vi "MDO_video_analyzer.vi"() -> ()   [LabVIEW 2012]
uses:
  controls/Video_analizer_stats.ctl
  <vilib>/vision/Avi.llb/IMAQ AVI2 Codec Path.ctl
panel:
  out "Image":T1(plugin-control) caption="300В-пуск-1.avi"
  in  "Save image":bool
  in  "Enum":enum16{"Осциллограммы", "ВАХ"}(ring)=enum."ВАХ"
  in  "Load DAQ Data":bool
  in  "Load Video":bool
  in  "Frame Forward":bool
  in  "Frame Back":bool
  in  "Settings Button":bool
  in  "Play Button":bool
  in  "Slide":u32(slide) max=200 scale=0.0..200.0
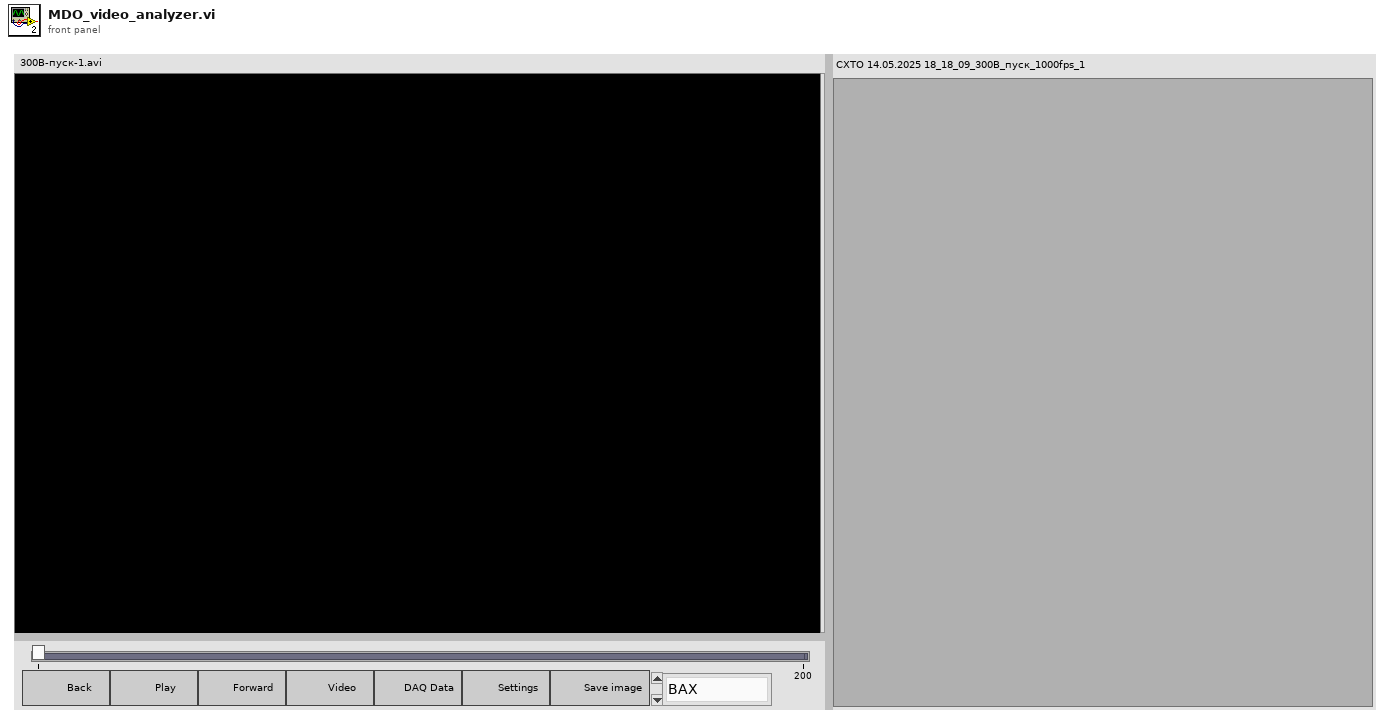
[diagram p1: front panel]
types:
  T1 = typedef "IMAQ Image.ctl" = refnum<image>
  T2 = typedef "Video_analizer_stats.ctl" = enum16{"Stop", "Initializ", "Play", "Pause", "Forward", "Back", "Slide", "Update UI", "Load video", "Load DAQ data", "Save image"}
  T3 = enum8{"Enabled", "Disabled", "Disabled and Grayed Out"}
  T4 = typedef "IMAQ AVI2 Refnum.ctl" = refnum<k20>
  T5 = typedef "IMAQ AVI2 Codec Path.ctl" = u32
  T6 = typedef "Image Type" = u32
  T7 = cluster{"Width":u32, "Height":u32, "Frames Per Second":u32, "Codec":string, "Has Data":bool}
  T8 = typedef "Video_analizer_settings.ctl" = cluster{"Current_shift":dbl, "Video_shift":dbl, "CurrentY_offset":dbl, "VoltageY_offset":dbl, "FIR_enable":bool, "Cutof_freq":dbl, "Order":u32}
  T9 = enum32{"invalid app kind", "Development System", "Run Time System", "Student Edition", "Embedded LabVIEW", "Evaluation", "Custom"}
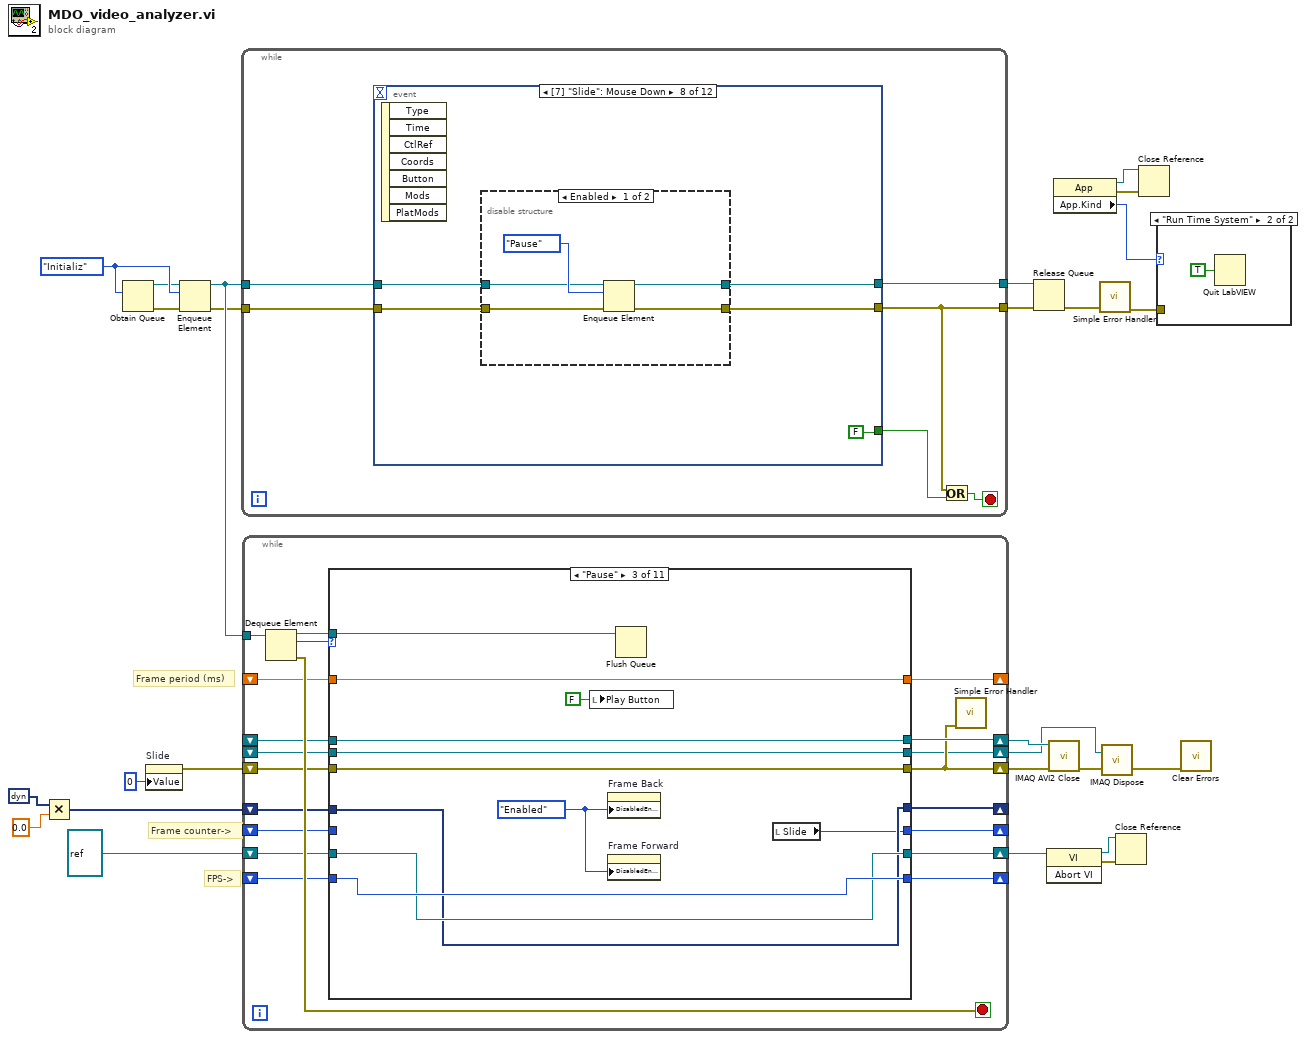
[diagram p0: block diagram]
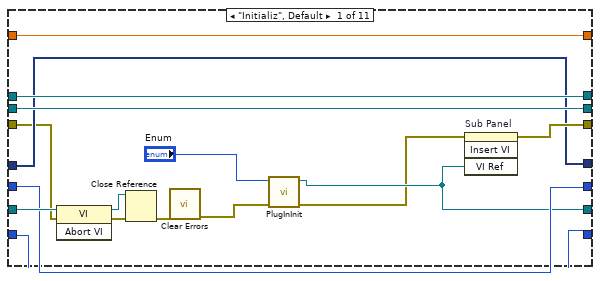
[diagram p3: hidden frame]
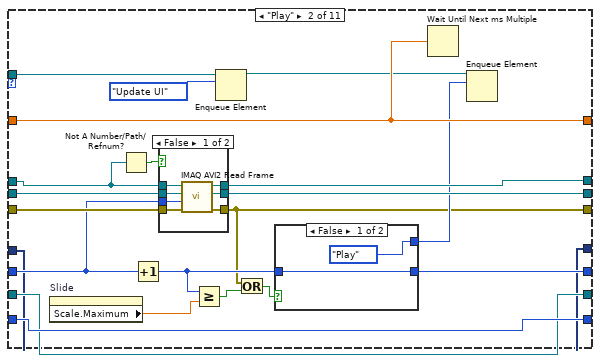
[diagram p4: hidden frame]
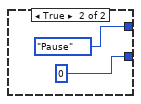
[diagram p6: hidden frame]
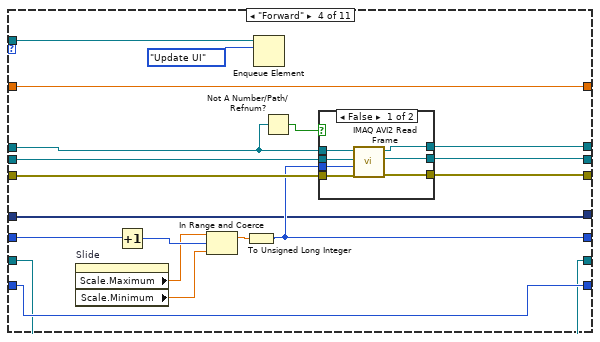
[diagram p7: hidden frame]
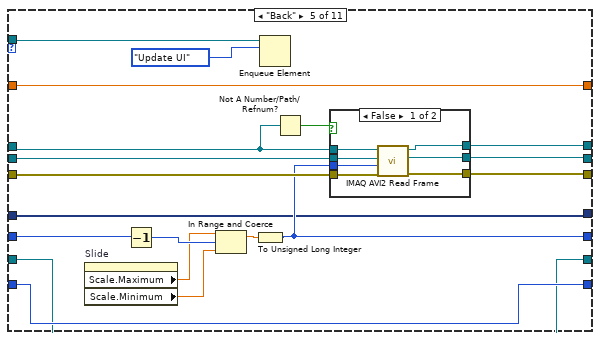
[diagram p9: hidden frame]
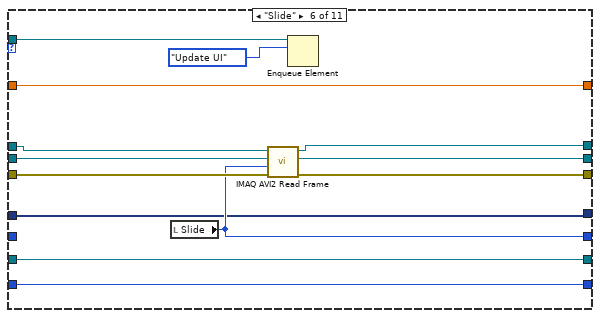
[diagram p11: hidden frame]
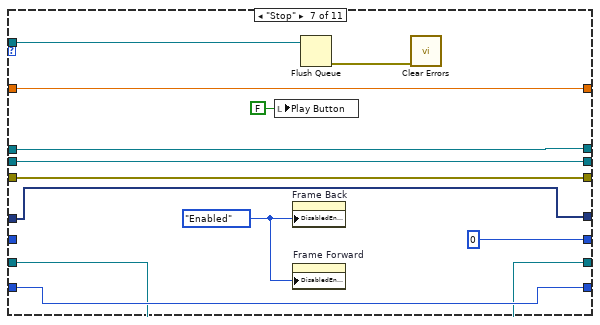
[diagram p12: hidden frame]
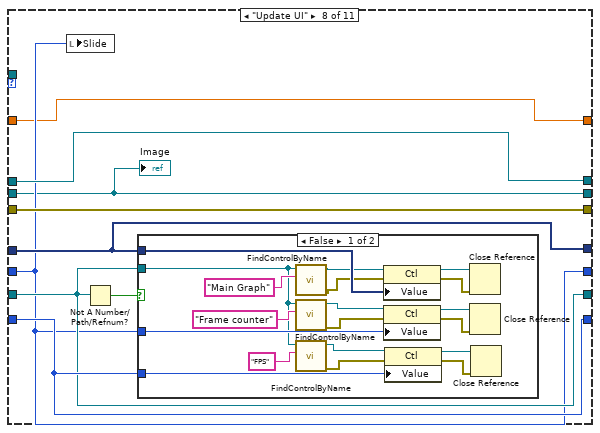
[diagram p13: hidden frame]
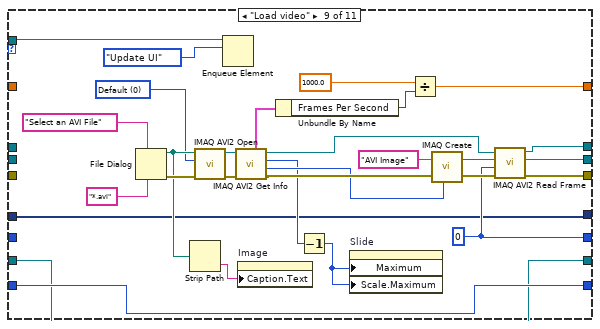
[diagram p15: hidden frame]
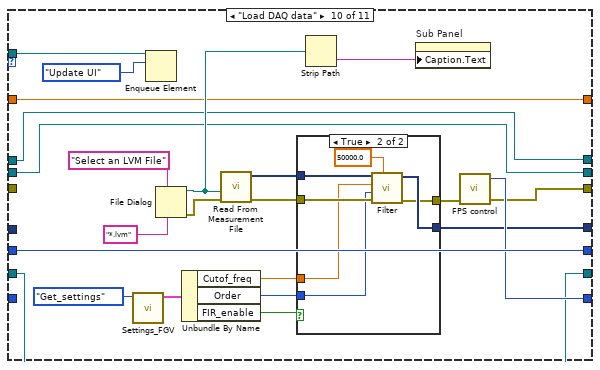
[diagram p16: hidden frame]
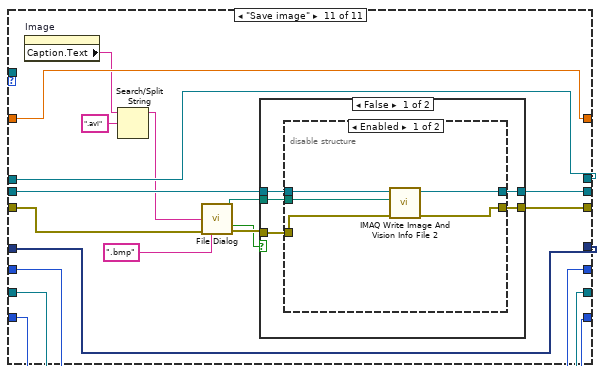
[diagram p18: hidden frame]
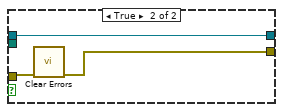
[diagram p20: hidden frame]
diagram:
  w15 = Video_analizer_stats."Initializ" ("video_analyzer_states")
  # "FPS->"
  # "Frame counter->"
  # "Frame period (ms)"
  n1 = Multiply(x=dynamicdata [{"t0"=timestamp(0 s since 1904-01-01), "dt"=1.0, "Y"=array[10000 elements], "attributes"=variant("NI_ChannelName"=variant(string "Voltage"), "NI_ExpIsRelativeTime"=variant(bool TRUE), "NI_ExpStartTimeStamp"=variant(timestamp timestamp(3710244565.071289 s since 1904-01-01)), "NI_ExpTimeStamp"=variant(timestamp timestamp(0 s since 1904-01-01)), "NI_ExpXDimension"=variant(string "t"))}, {"t0"=timestamp(0 s since 1904-01-01), "dt"=1.0, "Y"=array[10000 elements], "attributes"=variant("NI_ChannelName"=variant(string "Current"), "NI_ExpIsRelativeTime"=variant(bool TRUE), "NI_ExpStartTimeStamp"=variant(timestamp timestamp(3710244565.071289 s since 1904-01-01)), "NI_ExpTimeStamp"=variant(timestamp timestamp(0 s since 1904-01-01)), "NI_ExpXDimension"=variant(string "t"))}] ("Main Graph 2"), y=0.0) -> (x*y=w1:dynamicdata)
  n2 = Obtain Queue(element data type=w15) -> (queue out=w14:refnum<queue>, error out=w13:errorcluster)  [unwired: 4 in, 1 out]
  n3 = property on="Slide" class="Slide (strict)"("Value"=u32 0 ("Slide")) -> (error out=w19:errorcluster)  [unwired: 2 in, 1 out]
  n4 = Enqueue Element(queue=w14, element=w15, error in (no error)=w13) -> (queue out=w17:refnum<queue>, error out=w16:errorcluster)  [unwired: 1 in, 1 out]
  n5 = while {
    tunnel: w17 -> [w32]
    tunnel: w16 -> [w31]
    tunnel: [w28] -> w26
    tunnel: [w30] -> w25
    stop <- w29 stop-if-true
    n6 = event shown="[7] \"Slide\": Mouse Down" {
      selector: _ -> [_ _ _ _ _ _ _ _ _ _ _ _]
      dyn-events: _ -> [_ _ _ _ _ _ _ _ _ _ _ _]
      timeout: _ -> [_ _ _ _ _ _ _ _ _ _ _ _]
      tunnel: w32 -> [w35 w43 w51 w56 w62 w69 w74 w82 w91 w96 w109 w117]
      tunnel: w31 -> [w34 w42 w52 w57 w63 w68 w77 w81 w92 w102 w110 w119]
      tunnel: [w34 w41 w49 w54 w60 w66 w76 w80 w89 w97 w110 w113] -> w28
      tunnel: [w35 w40 w50 w55 w61 w67 w73 w79 w90 w95 w109 w115] -> w30
      tunnel: [FALSE FALSE FALSE FALSE FALSE FALSE FALSE ("T button?") FALSE FALSE FALSE w105 FALSE] -> w27
      event Timeout {
        n7 = event-data() -> ()  [unwired: 1 in, 2 out]
      }
      event "Play Button": Value Change {
        n8 = event-data() -> ()  [unwired: 1 in, 5 out]
        n9 = case shown="True" "Play Button" {
          tunnel: [Video_analizer_stats."Pause" ("element") Video_analizer_stats."Play" ("element")] -> w37
          tunnel: [T3."Enabled" ("Disabled") T3."Disabled" ("Disabled")] -> w36
          frame False {
          }
          frame True {
          }
        }
        n10 = property on="Frame Back" class="Bool"("DisabledEnum"=w36) -> ()  [unwired: 2 in, 2 out]
        n11 = property on="Frame Forward" class="Bool"("DisabledEnum"=w36) -> ()  [unwired: 2 in, 2 out]
        n12 = Enqueue Element(queue=w43, element=w37, error in (no error)=w42) -> (queue out=w40:refnum<queue>, error out=w41:errorcluster)  [unwired: 1 in, 1 out]
      }
      event "Frame Back": Value Change {
        n13 = event-data() -> ()  [unwired: 1 in, 5 out]
        n14 = Enqueue Element(queue=w51, element=Video_analizer_stats."Back", error in (no error)=w52) -> (queue out=w50:refnum<queue>, error out=w49:errorcluster)  [unwired: 1 in, 1 out]
      }
      event "Frame Forward": Value Change {
        n15 = event-data() -> ()  [unwired: 1 in, 5 out]
        n16 = Enqueue Element(queue=w56, element=Video_analizer_stats."Forward", error in (no error)=w57) -> (queue out=w55:refnum<queue>, error out=w54:errorcluster)  [unwired: 1 in, 1 out]
      }
      event "Load Video": Value Change {
        n17 = event-data() -> ()  [unwired: 1 in, 5 out]
        n18 = Enqueue Element(queue=w62, element=Video_analizer_stats."Load video", error in (no error)=w63) -> (queue out=w61:refnum<queue>, error out=w60:errorcluster)  [unwired: 1 in, 1 out]
      }
      event "Load DAQ Data": Value Change {
        n19 = event-data() -> ()  [unwired: 1 in, 5 out]
        n20 = Enqueue Element(queue=w69, element=Video_analizer_stats."Load DAQ data", error in (no error)=w68) -> (queue out=w67:refnum<queue>, error out=w66:errorcluster)  [unwired: 1 in, 1 out]
      }
      event "Save image": Value Change {
        n21 = event-data() -> ()  [unwired: 1 in, 5 out]
        n22 = Enqueue Element(queue=w74, element=Video_analizer_stats."Save image", error in (no error)=w77) -> (queue out=w73:refnum<queue>, error out=w76:errorcluster)  [unwired: 1 in, 1 out]
      }
      event "Slide": Mouse Down {
        n23 = event-data() -> ()  [unwired: 1 in, 7 out]
        n24 = disable-structure shown="Enabled" {
          disable-tunnel: w82 -> [w86 _]
          disable-tunnel: w81 -> [w85 _]
          disable-tunnel: [w84 _] -> w80
          disable-tunnel: [w83 _] -> w79
          frame Enabled {
            n25 = Enqueue Element(queue=w86, element=Video_analizer_stats."Pause", error in (no error)=w85) -> (queue out=w83:refnum<queue>, error out=w84:errorcluster)  [unwired: 1 in, 1 out]
          }
          frame Disabled {
          }
        }
      }
      event "Slide": Value Change {
        n26 = event-data() -> ()  [unwired: 1 in, 6 out]
        n27 = Enqueue Element(queue=w91, element=Video_analizer_stats."Slide", error in (no error)=w92) -> (queue out=w90:refnum<queue>, error out=w89:errorcluster)  [unwired: 1 in, 1 out]
      }
      event "Settings Button": Value Change {
        n28 = event-data() -> ()  [unwired: 1 in, 5 out]
        n29 = call "Settings_FGV.vi"("error in (no error)"=w102, "State"=enum16{"Get_settings", "Set_settings"}."Set_settings") -> ("error out"=w94:errorcluster)  [unwired: 8 in, 1 out]
        n30 = Enqueue Element(queue=w96, element=Video_analizer_stats."Initializ", error in (no error)=w94) -> (queue out=w100:refnum<queue>, error out=w99:errorcluster)  [unwired: 1 in, 1 out]
        n31 = Enqueue Element(queue=w100, element=Video_analizer_stats."Update UI", error in (no error)=w99) -> (queue out=w95:refnum<queue>, error out=w97:errorcluster)  [unwired: 1 in, 1 out]
      }
      event Panel Close? {
        n32 = event-data() -> ()  [unwired: 1 in, 3 out]
        n33 = Two Button Dialog(message="Вы действительно хотите закрыть программу?", 1:"Нет" ("F button name (\"Cancel\")"), 2:"Да" ("T button name (\"OK\")")) -> (T button?=w105:bool)
        n34 = event-data("Discard?"=TRUE) -> ()  [unwired: 1 in, 1 out]
      }
      event "Enum": Value Change {
        n35 = event-data() -> ()  [unwired: 1 in, 5 out]
        n36 = Enqueue Element(queue=w117, element=Video_analizer_stats."Initializ", error in (no error)=w119) -> (queue out=w116:refnum<queue>, error out=w114:errorcluster)  [unwired: 1 in, 1 out]
        n37 = Enqueue Element(queue=w116, element=Video_analizer_stats."Update UI", error in (no error)=w114) -> (queue out=w115:refnum<queue>, error out=w113:errorcluster)  [unwired: 1 in, 1 out]
      }
    }
    n38 = Or(x=w28, y=w27) -> (x .or. y?=w29:bool)
  }
  n39 = while {
    tunnel: w17 -> [w140]
    shift-right: [w129] -> w20
    shift-left: _ -> [w133]
    shift-right: [w136] -> w21
    shift-left: _ -> [w132]
    shift-right: [w128] -> _
    shift-left: _ -> [w131]
    shift-right: [w135] -> w22
    shift-left: w19 -> [w134]
    shift-right: [w126] -> _
    shift-left: _ -> [w130]
    shift-right: [w125] -> _
    shift-left: _ -> [w127]
    shift-right: [w124] -> w10
    shift-left: refnum<vi> refnum -> [w123]
    shift-right: [w122] -> _
    shift-left: w1 -> [w121]
    stop <- w138 stop-if-true
    n40 = Dequeue Element(queue=w140) -> (queue out=w137:refnum<queue>, element=w139:T2, error out=w138:errorcluster)  [unwired: 2 in, 1 out]
    n41 = case shown="\"Pause\"" w139 {
      tunnel: w137 -> [_ w167 w202 w207 w236 w261 w283 _ w317 w353 _]
      tunnel: [w156 w175 w198 w216 w241 w268 w279 w286 w322 w359 w390] -> w129
      tunnel: [w155 w176 w199 w215 w240 w269 w278 w294 w324 w360 w388] -> w136
      tunnel: [w154 w168 w200 w214 w239 w267 w282 w287 w331 w361 w380] -> w128
      tunnel: [w151 w159 w197 w217 w242 w272 w280 w293 w326 w356 w389] -> w135
      tunnel: w134 -> [w143 w177 w197 w220 w245 w273 w280 w293 _ _ w384]
      tunnel: w133 -> [w156 w174 w198 w221 w246 w271 w279 w286 _ w359 w391]
      tunnel: w132 -> [w155 w158 w199 w204 w233 w270 w278 w294 _ w360 w388]
      tunnel: w131 -> [w154 w168 w200 w214 w239 w267 w282 w287 _ w361 w380]
      tunnel: [w146 w171 w192 w210 w243 w266 u32 0 ("Slide") w288 w327 w358 w386] -> w126
      tunnel: w130 -> [w146 w173 _ w218 w244 _ _ w288 _ w358 w386]
      tunnel: [w153 w169 w195 w209 w238 w265 w281 w290 w319 w357 w379] -> w125
      tunnel: w127 -> [w153 w169 w195 w209 w238 w265 w281 w290 w319 _ w379]
      tunnel: [w145 w164 w194 w206 w235 w263 w275 w289 w316 w355 w378] -> w124
      tunnel: w123 -> [w150 w164 w194 w206 w235 w263 w275 w289 w316 w355 w378]
      tunnel: [w147 w163 w193 w205 w234 w262 w274 w291 w315 w350 w387] -> w122
      tunnel: w121 -> [w147 w163 w193 w205 w234 w262 w274 w291 w315 _ w387]
      frame "Initializ", Default {
        n42 = invoke class="VI" method="Abort VI"(reference=w150, error in=w143) -> (reference out=w148:refnum<vi>, error out=w149:errorcluster)  [unwired: 1 in, 1 out]
        n43 = Close Reference(reference=w148, error in (no error)=w149) -> (error out=w142:errorcluster)
        n44 = call <vilib>:"Clear Errors.vi"("error in (no error)"=w142) -> ("error out"=w141:errorcluster)  [unwired: 6 in]
        n45 = call "PlugInInit.vi"("error in (no error)"=w141, "Enum"="Enum") -> ("error out"=w144:errorcluster, "PlugIn_VI_out"=w145:refnum<vi>)  [unwired: 8 in]
        n46 = invoke on="Sub Panel" class="SubPanel" method="Insert VI"(error in=w144, "VI Ref"=w145) -> (error out=w151:errorcluster)  [unwired: 2 in, 3 out]
      }
      frame "Play" {
        n47 = property on="Slide" class="Slide (strict)"() -> ("Scale.Maximum"=w172:dbl)  [unwired: 2 in, 2 out]
        n48 = Not A Number/Path/Refnum?(number/path/refnum=w158) -> (NaN/Path/Refnum?=w157:bool)
        n49 = Increment(x=w173) -> (x+1=w170:u32)
        n50 = case shown="False" w157 {
          tunnel: w177 -> [w184 w185]
          tunnel: [w183 w187] -> w176
          tunnel: [w182 w186] -> w175
          tunnel: w174 -> [w181 w186]
          tunnel: w173 -> [w180 _]
          tunnel: [w179 w185] -> w159
          tunnel: w158 -> [w178 w187]
          frame False {
            n51 = call "IMAQ AVI2 Read Frame"("error in (no error)"=w184, "Frame Number"=w180, "Image"=w181, "AVI Refnum"=w178) -> ("error out"=w179:errorcluster, "Image Out"=w182:T1, "AVI Refnum (duplicate)"=w183:T4)  [unwired: 5 out]
          }
          frame True {
          }
        }
        n52 = Greater Or Equal?(x=w170, y=w172) -> (x >= y?=w161:bool)
        n53 = Enqueue Element(queue=w167, element=Video_analizer_stats."Update UI") -> (queue out=w166:refnum<queue>)  [unwired: 2 in, 2 out]
        n54 = Or(x=w159, y=w161) -> (x .or. y?=w160:bool)
        n55 = case shown="False" w160 {
          tunnel: [w189 u32 0] -> w171
          tunnel: w170 -> [w189 _]
          tunnel: [Video_analizer_stats."Play" ("element") Video_analizer_stats."Pause" ("element")] -> w162
          frame False {
          }
          frame True {
          }
        }
        n56 = Wait Until Next ms Multiple(millisecond multiple=w168) -> ()  [unwired: 1 out]
        n57 = Enqueue Element(queue=w166, element=w162) -> ()  [unwired: 2 in, 3 out]
      }
      frame "Pause" {
        w196 = T3."Enabled" ("Disabled")
        n58 = local write "Play Button"(FALSE ("Play Button")) -> ()
        n59 = property on="Frame Back" class="Bool"("DisabledEnum"=w196) -> ()  [unwired: 2 in, 2 out]
        n60 = property on="Frame Forward" class="Bool"("DisabledEnum"=w196) -> ()  [unwired: 2 in, 2 out]
        n61 = Flush Queue(queue=w202) -> ()  [unwired: 1 in, 3 out]
        n62 = local read "Slide"() -> (w192:u32)
      }
      frame "Forward" {
        n63 = property on="Slide" class="Slide (strict)"() -> ("Scale.Maximum"=w213:dbl, "Scale.Minimum"=w212:dbl)  [unwired: 2 in, 2 out]
        n64 = Increment(x=w218) -> (x+1=w219:u32)
        n65 = In Range and Coerce(upper limit=w213, x=w219, lower limit=w212) -> (coerced(x)=w211:dbl)  [unwired: 1 out]
        n66 = To Unsigned Long Integer(number=w211) -> (unsigned 32bit integer=w210:u32)
        n67 = Enqueue Element(queue=w207, element=Video_analizer_stats."Update UI") -> ()  [unwired: 2 in, 3 out]
        n68 = Not A Number/Path/Refnum?(number/path/refnum=w204) -> (NaN/Path/Refnum?=w203:bool)
        n69 = case shown="False" w203 {
          tunnel: w204 -> [w228 w231]
          tunnel: w221 -> [w227 w230]
          tunnel: w220 -> [w226 w229]
          tunnel: [w225 w229] -> w217
          tunnel: [w224 w230] -> w216
          tunnel: [w223 w231] -> w215
          tunnel: w210 -> [w222 _]
          frame False {
            n70 = call "IMAQ AVI2 Read Frame"("error in (no error)"=w226, "Frame Number"=w222, "Image"=w227, "AVI Refnum"=w228) -> ("error out"=w225:errorcluster, "Image Out"=w224:T1, "AVI Refnum (duplicate)"=w223:T4)  [unwired: 5 out]
          }
          frame True {
          }
        }
      }
      frame "Back" {
        n71 = property on="Slide" class="Slide (strict)"() -> ("Scale.Maximum"=w249:dbl, "Scale.Minimum"=w248:dbl)  [unwired: 2 in, 2 out]
        n72 = Decrement(x=w244) -> (x-1=w250:u32)
        n73 = In Range and Coerce(upper limit=w249, x=w250, lower limit=w248) -> (coerced(x)=w247:dbl)  [unwired: 1 out]
        n74 = To Unsigned Long Integer(number=w247) -> (unsigned 32bit integer=w243:u32)
        n75 = Enqueue Element(queue=w236, element=Video_analizer_stats."Update UI") -> ()  [unwired: 2 in, 3 out]
        n76 = Not A Number/Path/Refnum?(number/path/refnum=w233) -> (NaN/Path/Refnum?=w232:bool)
        n77 = case shown="False" w232 {
          tunnel: w233 -> [w257 w260]
          tunnel: w246 -> [w256 w259]
          tunnel: w245 -> [w255 w258]
          tunnel: w243 -> [w254 _]
          tunnel: [w253 w258] -> w242
          tunnel: [w252 w259] -> w241
          tunnel: [w251 w260] -> w240
          frame False {
            n78 = call "IMAQ AVI2 Read Frame"("error in (no error)"=w255, "Frame Number"=w254, "Image"=w256, "AVI Refnum"=w257) -> ("error out"=w253:errorcluster, "Image Out"=w252:T1, "AVI Refnum (duplicate)"=w251:T4)  [unwired: 5 out]
          }
          frame True {
          }
        }
      }
      frame "Slide" {
        n79 = local read "Slide"() -> (w266:u32)
        n80 = call "IMAQ AVI2 Read Frame"("error in (no error)"=w273, "Frame Number"=w266, "Image"=w271, "AVI Refnum"=w270) -> ("error out"=w272:errorcluster, "Image Out"=w268:T1, "AVI Refnum (duplicate)"=w269:T4)  [unwired: 5 out]
        n81 = Enqueue Element(queue=w261, element=Video_analizer_stats."Update UI") -> ()  [unwired: 2 in, 3 out]
      }
      frame "Stop" {
        w284 = T3."Enabled" ("Disabled")
        n82 = local write "Play Button"(FALSE ("Play Button")) -> ()
        n83 = property on="Frame Back" class="Bool"("DisabledEnum"=w284) -> ()  [unwired: 2 in, 2 out]
        n84 = property on="Frame Forward" class="Bool"("DisabledEnum"=w284) -> ()  [unwired: 2 in, 2 out]
        n85 = Flush Queue(queue=w283) -> (error out=w276:errorcluster)  [unwired: 1 in, 2 out]
        n86 = call <vilib>:"Clear Errors.vi"("error in (no error)"=w276) -> ()  [unwired: 6 in, 1 out]
      }
      frame "Update UI" {
        n87 = local write "Slide"(w288) -> ()
        n88 = Not A Number/Path/Refnum?(number/path/refnum=w289) -> (NaN/Path/Refnum?=w292:bool)
        n89 = case shown="False" w292 {
          tunnel: w289 -> [w298 _]
          tunnel: w291 -> [w307 _]
          tunnel: w288 -> [w306 _]
          tunnel: w290 -> [w305 _]
          frame False {
            n90 = call "FindControlByName.vi"("Control_name"="Main Graph" ("control name"), "VI Refnum"=w298) -> ("error out"=w303:errorcluster, "reference out"=w302:refnum<vi>)  [unwired: 8 in]
            n91 = call "FindControlByName.vi"("Control_name"="Frame counter" ("control name"), "VI Refnum"=w298) -> ("error out"=w300:errorcluster, "reference out"=w299:refnum<vi>)  [unwired: 8 in]
            n92 = call "FindControlByName.vi"("Control_name"="FPS" ("control name"), "VI Refnum"=w298) -> ("error out"=w296:errorcluster, "reference out"=w295:refnum<vi>)  [unwired: 8 in]
            n93 = property class="Ctl"(reference=w302, error in=w303, "Value"=w307) -> (reference out=w313:refnum<vi>, error out=w312:errorcluster)
            n94 = property class="Ctl"(reference=w299, error in=w300, "Value"=w306) -> (reference out=w309:refnum<vi>, error out=w311:errorcluster)
            n95 = property class="Ctl"(reference=w295, error in=w296, "Value"=w305) -> (reference out=w308:refnum<vi>, error out=w310:errorcluster)
            n96 = Close Reference(reference=w313, error in (no error)=w312) -> ()  [unwired: 1 out]
            n97 = Close Reference(reference=w309, error in (no error)=w311) -> ()  [unwired: 1 out]
            n98 = Close Reference(reference=w308, error in (no error)=w310) -> ()  [unwired: 1 out]
          }
          frame True {
          }
        }
        "Image" <- w286
      }
      frame "Load video" {
        w314 = T5 0 items=["Default", "System", "Built in Vision"] ("Codec Source")
        w327 = u32 0
        n99 = File Dialog(6:"*.avi" ("pattern"), 7:"Select an AVI File" ("prompt")) -> (0:w338:errorcluster, 3:w321:path)  [unwired: 2 in, 5 out]
        n100 = Strip Path(path=w321) -> (name=w320:string)  [unwired: 1 out]
        n101 = call "IMAQ AVI2 Open"("error in (no error)"=w338, "Codec Source"=w314, "AVI File Path"=w321) -> ("error out"=w341:errorcluster, "AVI Refnum"=w340:T4)  [unwired: 7 out]
        n102 = Enqueue Element(queue=w317, element=Video_analizer_stats."Update UI") -> ()  [unwired: 2 in, 3 out]
        n103 = call "IMAQ AVI2 Get Info"("error in (no error)"=w341, "AVI Refnum"=w340) -> ("error out"=w336:errorcluster, "Image Type"=w335:T6, "Number of Frames"=w330:u32, "AVI Refnum (duplicate)"=w325:T4, "Frame Data"=w332:T7)  [unwired: 5 out]
        n104 = property on="Image" class="ImageControl"("Caption.Text"=w320) -> ()  [unwired: 2 in, 2 out]
        n105 = Unbundle By Name(w332) -> ("Frames Per Second"=w334:u32)
        n106 = Decrement(x=w330) -> (x-1=w329:u32)
        n107 = property on="Slide" class="Slide (strict)"("Maximum"=w329, "Scale.Maximum"=w329) -> ()  [unwired: 2 in, 2 out]
        n108 = Divide(x=1000.0, y=w334) -> (x/y=w331:dbl)
        n109 = call "IMAQ Create"("Image Name"="AVI Image", "Image Type"=w335, "error in (no error)"=w336) -> ("New Image"=w323:T1, "error out"=w328:errorcluster)  [unwired: 1 in, 1 out]
        n110 = call "IMAQ AVI2 Read Frame"("error in (no error)"=w328, "Frame Number"=w327, "Image"=w323, "AVI Refnum"=w325) -> ("error out"=w326:errorcluster, "Image Out"=w322:T1, "AVI Refnum (duplicate)"=w324:T4)  [unwired: 5 out]
      }
      frame "Load DAQ data" {
        n111 = call "Settings_FGV.vi"("State"=enum16{"Get_settings", "Set_settings"}."Get_settings") -> ("Settings"=w345:T8)  [unwired: 9 in, 1 out]
        n112 = Enqueue Element(queue=w353, element=Video_analizer_stats."Update UI") -> ()  [unwired: 2 in, 3 out]
        n113 = File Dialog(6:"*.lvm" ("pattern"), 7:"Select an LVM File" ("prompt")) -> (0:w363:errorcluster, 3:w362:path)  [unwired: 2 in, 5 out]
        n114 = Unbundle By Name(w345) -> ("Cutof_freq"=w343:dbl, "Order"=w344:u32, "FIR_enable"=w346:bool)
        n115 = call "Read From Measurement File"("error in (no error)"=w363, "Filename"=w362) -> ("error out"=w348:errorcluster, "Signals"=w351:dynamicdata)  [unwired: 4 in, 4 out]
        n116 = case shown="True" w346 {
          tunnel: w351 -> [w366 w374]
          tunnel: [w366 w373] -> w350
          tunnel: w348 -> [w367 w371]
          tunnel: [w367 w370] -> w347
          tunnel: w344 -> [_ w369]
          tunnel: w343 -> [_ w368]
          frame False {
          }
          frame True {
            n117 = call "Filter.vi"("sampling freq: fs"=50000.0, "error in (no error)"=w371, "order"=w369, "low cutoff freq: fl"=w368, "Data_in"=w374) -> ("error out"=w370:errorcluster, "Data_out"=w373:dynamicdata)  [unwired: 5 in]
          }
        }
        n118 = Strip Path(path=w362) -> (name=w352:string)  [unwired: 1 out]
        n119 = property on="Sub Panel" class="SubPnl"("Caption.Text"=w352) -> ()  [unwired: 2 in, 2 out]
        n120 = call "FPS control.vi"("error in (no error)"=w347) -> ("error out"=w356:errorcluster, "FPS out"=w357:u32)  [unwired: 3 in]
      }
      frame "Save image" {
        n121 = property on="Image" class="ImageControl"() -> ("Caption.Text"=w377:string)  [unwired: 2 in, 2 out]
        n122 = Search/Split String(string=w377, search string/char (-)=".avi") -> (substring before match=w376:string)  [unwired: 1 in, 2 out]
        n123 = call "File Dialog"("default name"=w376, "error in"=w384, "pattern (all files)"=".bmp") -> ("selected path"=w381:path, "cancelled"=w382:bool, "error out"=w383:errorcluster)  [unwired: 9 in, 1 out]
        n124 = case shown="False" w382 {
          tunnel: w391 -> [w396 w406]
          tunnel: w381 -> [w395 _]
          tunnel: w383 -> [w394 w405]
          tunnel: [w393 w406] -> w390
          tunnel: [w392 w404] -> w389
          frame False {
            n125 = disable-structure shown="Enabled" {
              disable-tunnel: w396 -> [w401 w403]
              disable-tunnel: w395 -> [w400 _]
              disable-tunnel: w394 -> [w399 w402]
              disable-tunnel: [w398 w403] -> w393
              disable-tunnel: [w397 w402] -> w392
              frame Enabled {
                n126 = call "IMAQ Write Image And Vision Info File 2"("error in (no error)"=w399, "File Path"=w400, "Image"=w401) -> ("error out"=w397:errorcluster, "Image Out (duplicate)"=w398:T1)  [unwired: 7 in]
              }
              frame Disabled {
              }
            }
          }
          frame True {
            n127 = call <vilib>:"Clear Errors.vi"("error in (no error)"=w405) -> ("error out"=w404:errorcluster)  [unwired: 6 in]
          }
        }
      }
    }
    n128 = call <vilib>:"Simple Error Handler.vi"("error in (no error)"=w135) -> ()  [unwired: 4 in, 5 out]
  }
  n129 = Release Queue(queue=w25, error in (no error)=w26) -> (error out=w24:errorcluster)  [unwired: 1 in, 2 out]
  n130 = invoke class="VI" method="Abort VI"(reference=w10) -> (reference out=w12:refnum<vi>, error out=w11:errorcluster)  [unwired: 2 in, 1 out]
  n131 = call "IMAQ AVI2 Close"("error in (no error)"=w22, "AVI Refnum"=w21) -> ("error out"=w23:errorcluster)  [unwired: 9 out]
  n132 = property class="App"() -> (reference out=w7:refnum<vi>, error out=w6:errorcluster, "App.Kind"=w5:T9)  [unwired: 2 in]
  n133 = call <vilib>:"Simple Error Handler.vi"("error in (no error)"=w24) -> ("error out"=w4:errorcluster)  [unwired: 4 in, 4 out]
  n134 = call "IMAQ Dispose"("Image"=w20, "error in (no error)"=w23) -> ("error out"=w8:errorcluster)  [unwired: 1 in, 3 out]
  n135 = Close Reference(reference=w12, error in (no error)=w11) -> ()  [unwired: 1 out]
  n136 = Close Reference(reference=w7, error in (no error)=w6) -> ()  [unwired: 1 out]
  n137 = case shown="\"Run Time System\"" w5 {
    tunnel: w4 -> [_ _]
    frame "Development System", Default {
    }
    frame "Run Time System" {
      n138 = Quit LabVIEW(quit? (T)=TRUE) -> ()
    }
  }
  n139 = call <vilib>:"Clear Errors.vi"("error in (no error)"=w8) -> ()  [unwired: 6 in, 1 out]
